vi "map_diag_piastre.vi"() -> ()   [LabVIEW 2015]
panel:
  in  "z inizio":bool
  in  "y inizio":bool
  in  "Positioning Done":bool
  in  "x inizio":bool
  in  "y inizio":bool
  in  "Positioning Done":bool
  in  "y inizio":bool
  in  "Positioning Done":bool
  in  "KILL":bool
  in  "PAUSE":bool
  in  "RESUME":bool
  in  "QUIT":bool
  in  "Positioning Done":bool
  in  "y inizio":bool
  in  "x inizio":bool
  in  "End":bool
  in  "zero z - end":bool
  in  "zero x - end":bool
  in  "zero y - end":bool
  out "output":string
  out "command":string
  in  "zero done":bool
  in  "zero z":bool
  in  "zero x":bool
  in  "zero y":bool
  # "Comandi di emergenza"
  # "Posiziono in zero"
  # "Vado al punto di partenza\nDiagonale Left Internal"
  # "Vado al punto di partenza\nDiagonale Right Internal"
  # "Vado al punto di partenza\nDiagonale Left External"
  # "Vado al punto di partenza\nDiagonale Right External"
  # "Ritorno a zero"
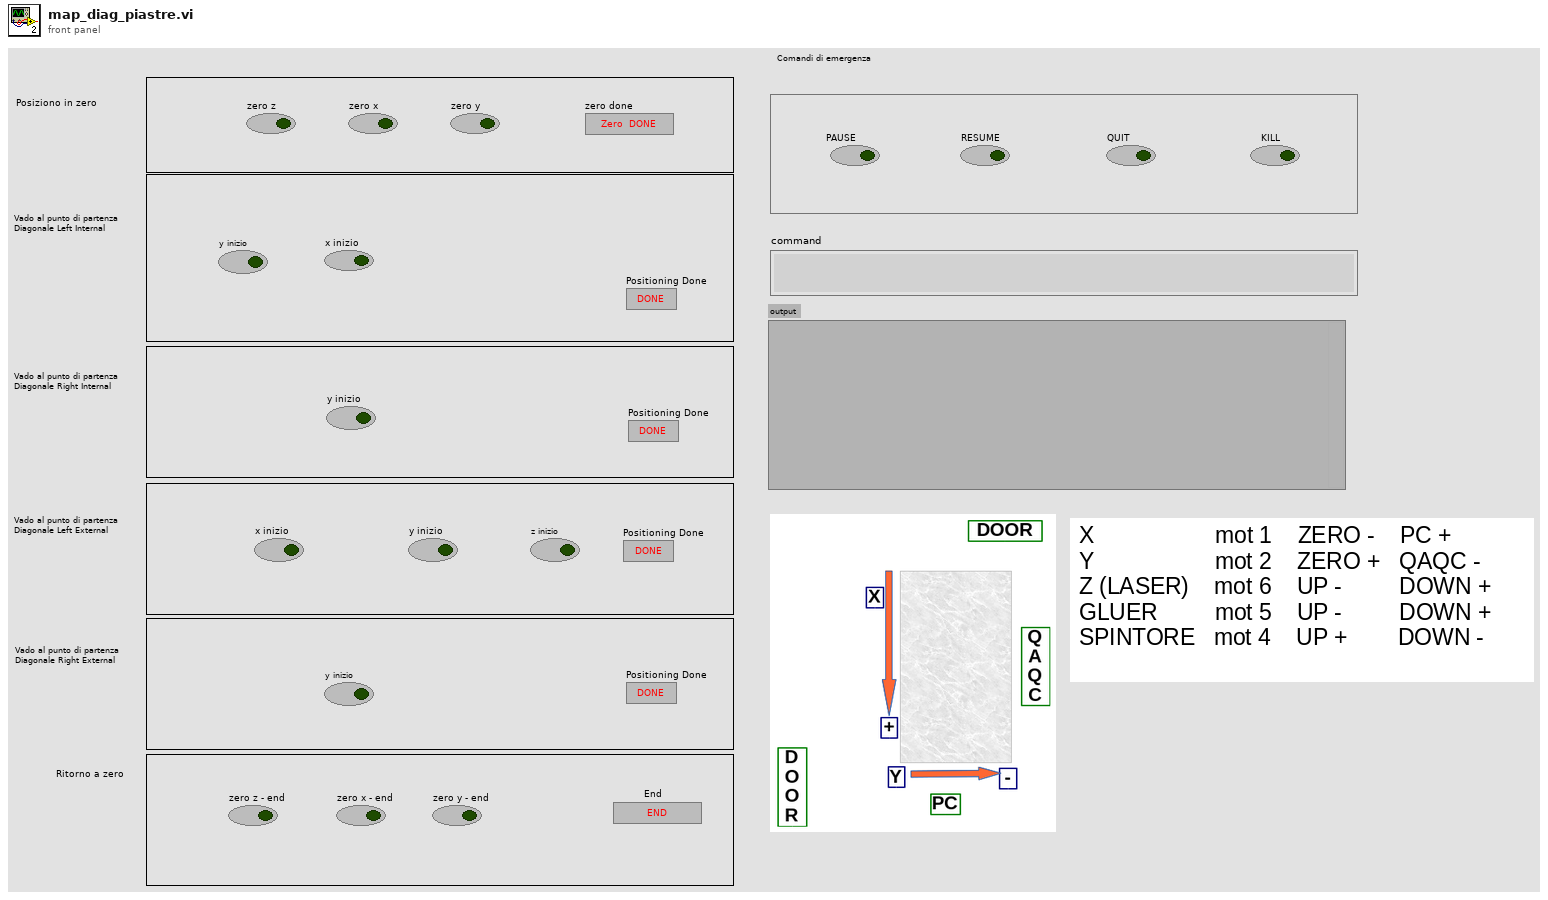
[diagram p1: front panel]
types:
  T1 = enum16{"open", "replace", "create", "open or create", "replace or create", "replace or create with confirmation"}
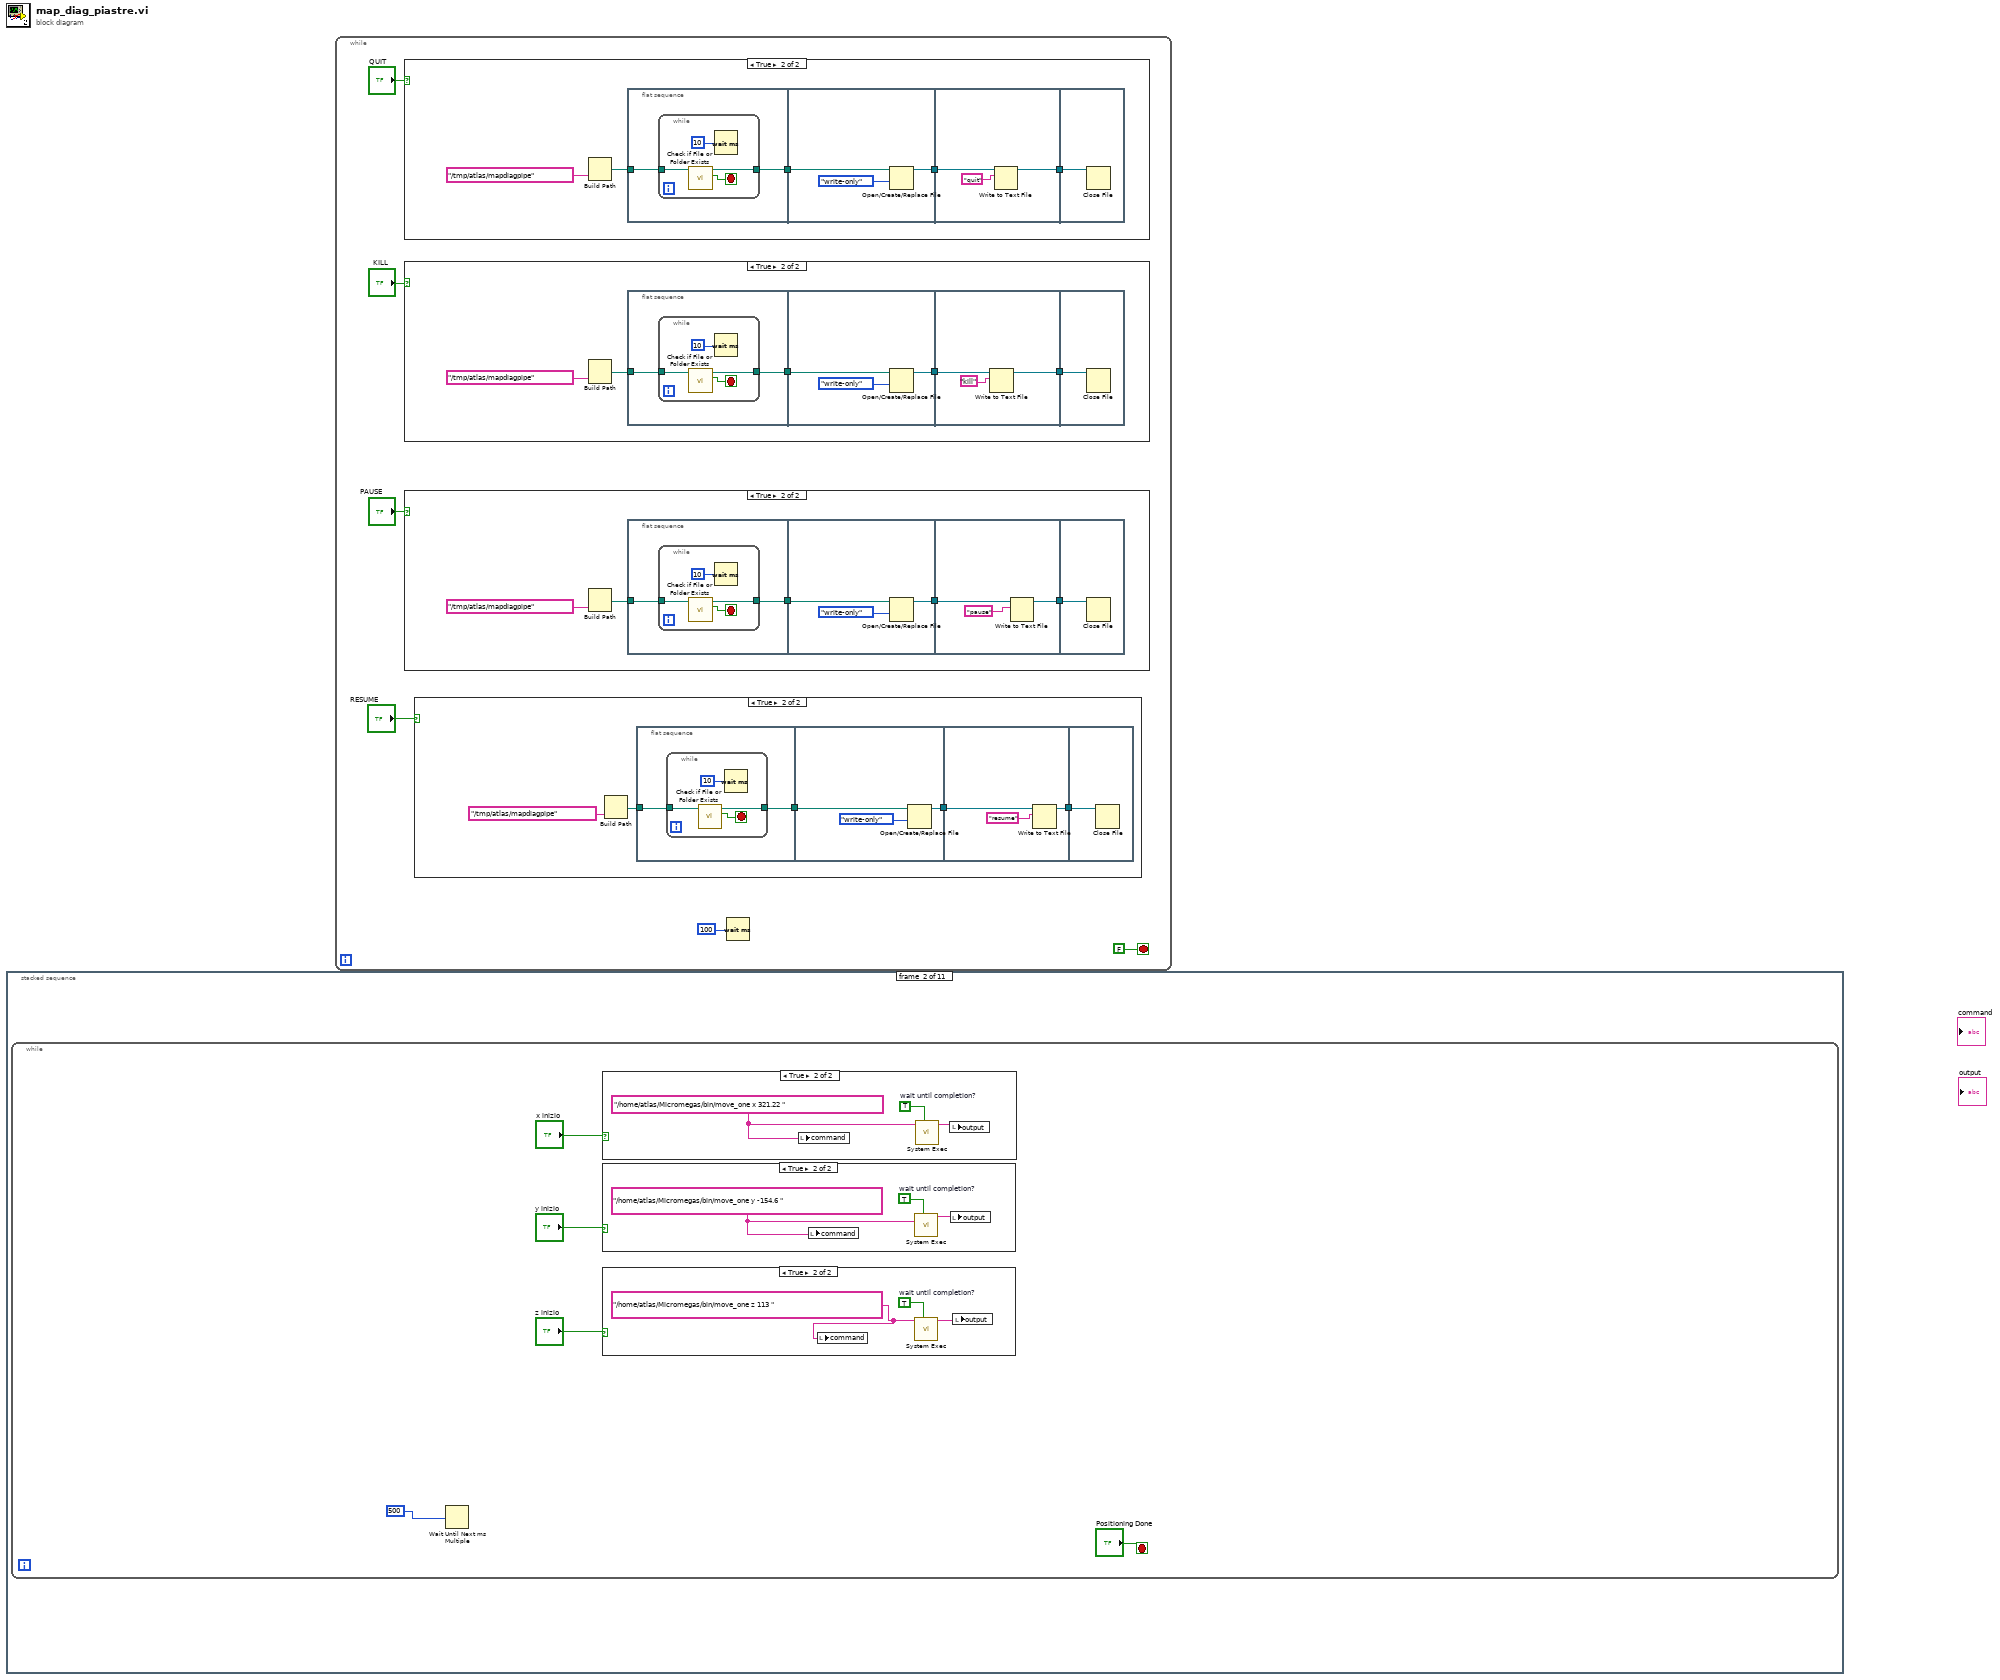
[diagram p0: block diagram]
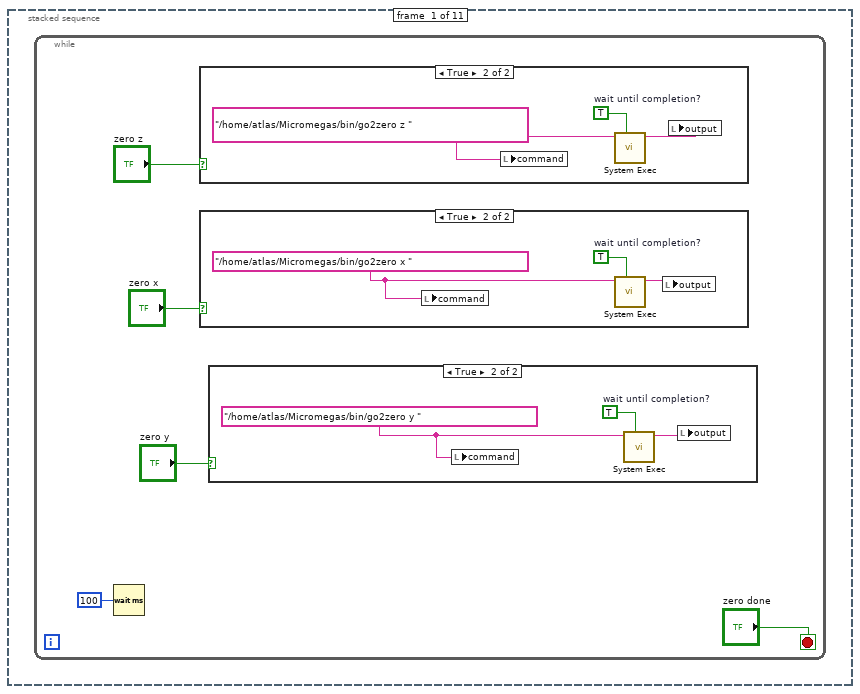
[diagram p6: hidden frame]
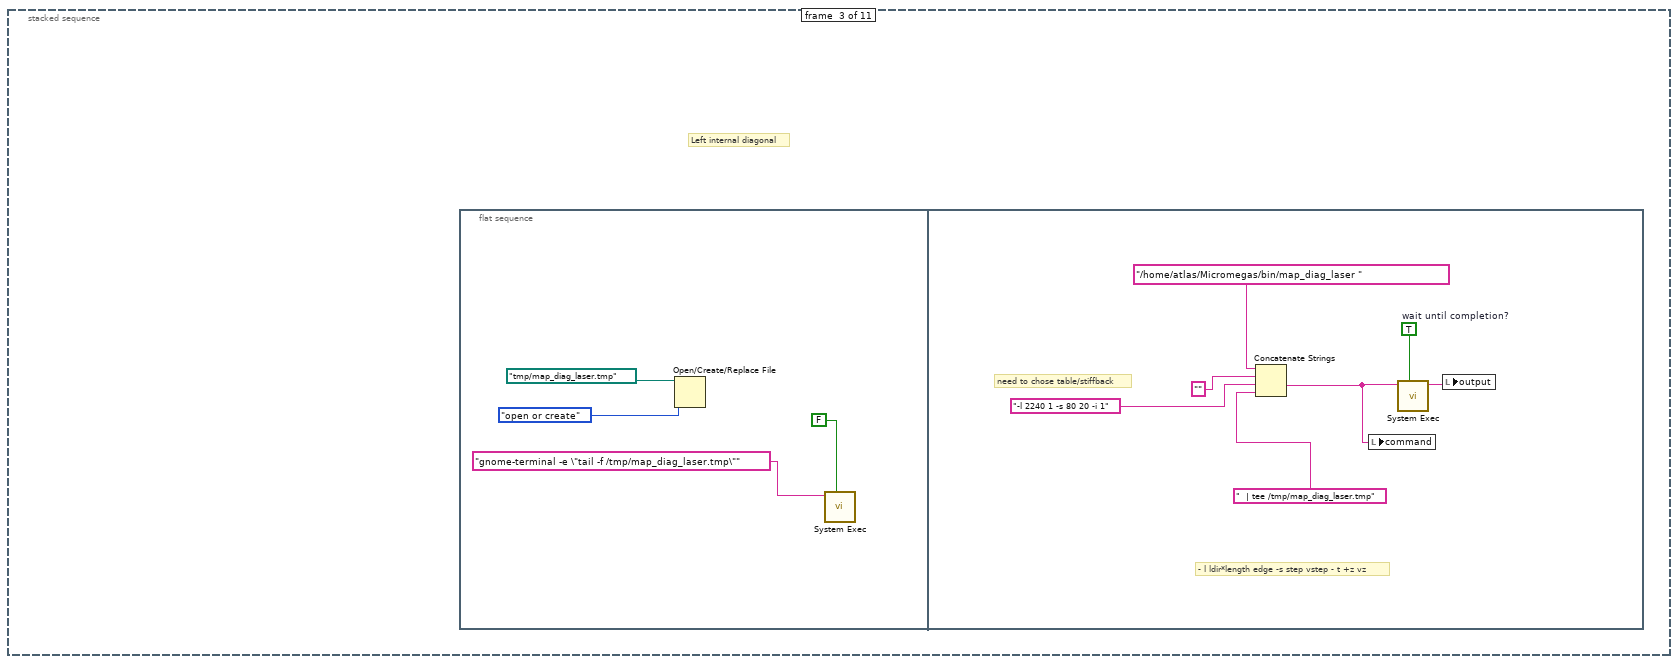
[diagram p13: hidden frame]
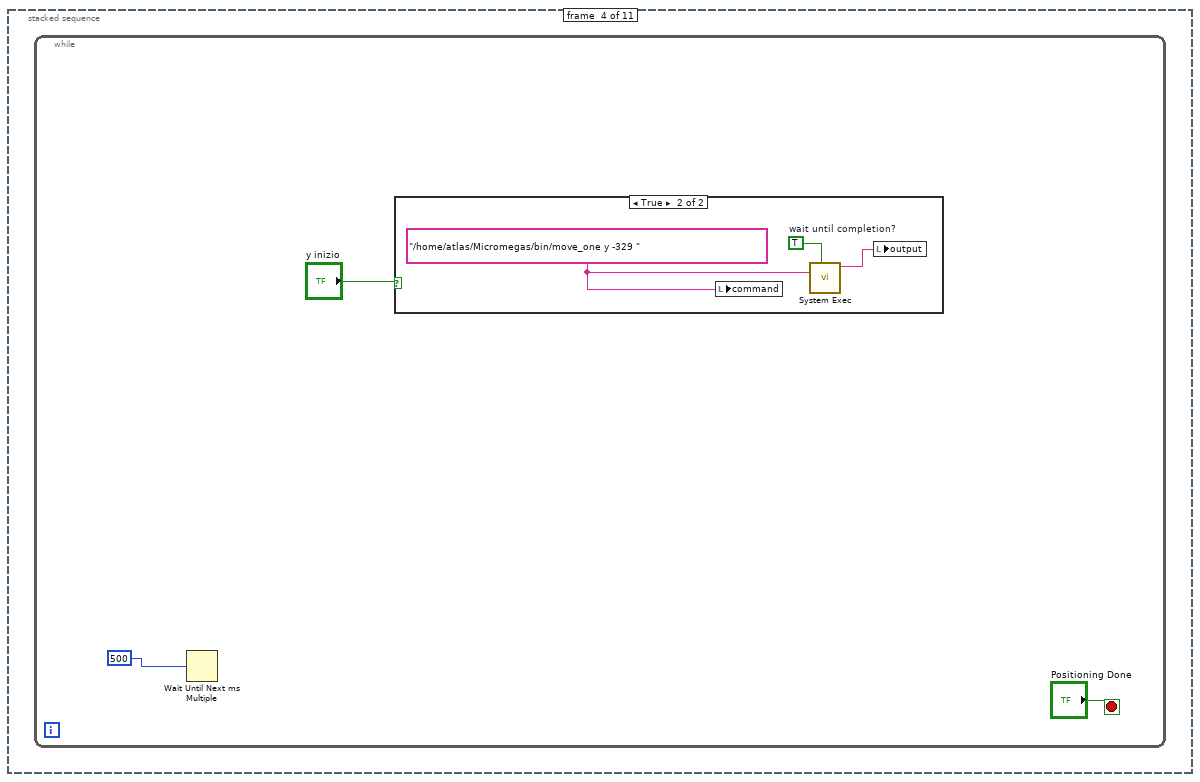
[diagram p14: hidden frame]
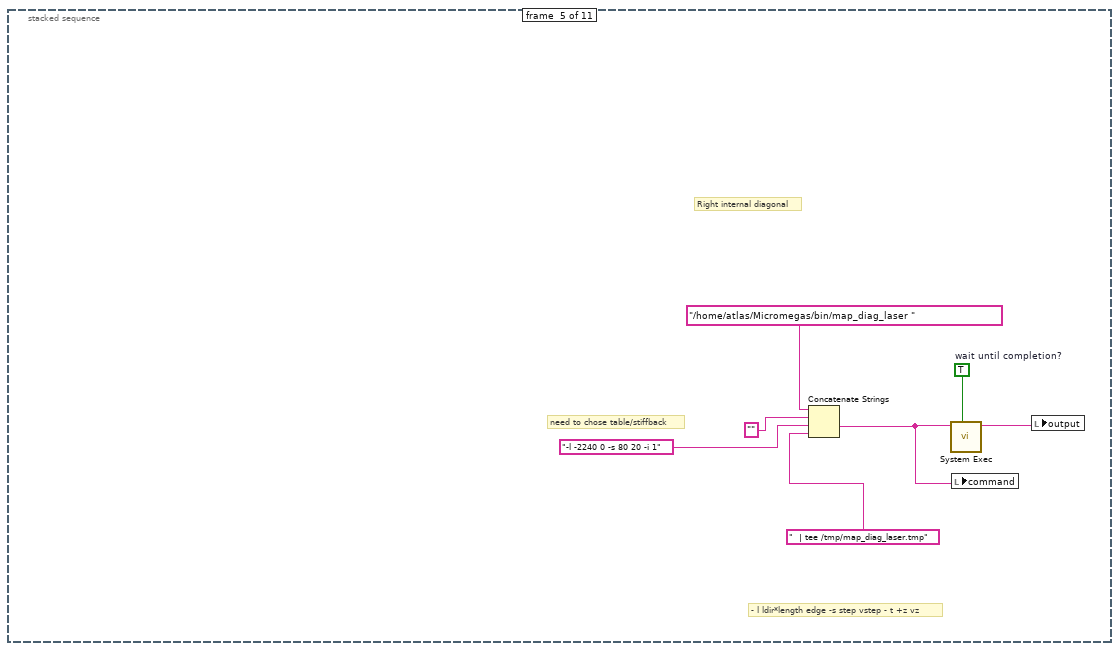
[diagram p16: hidden frame]
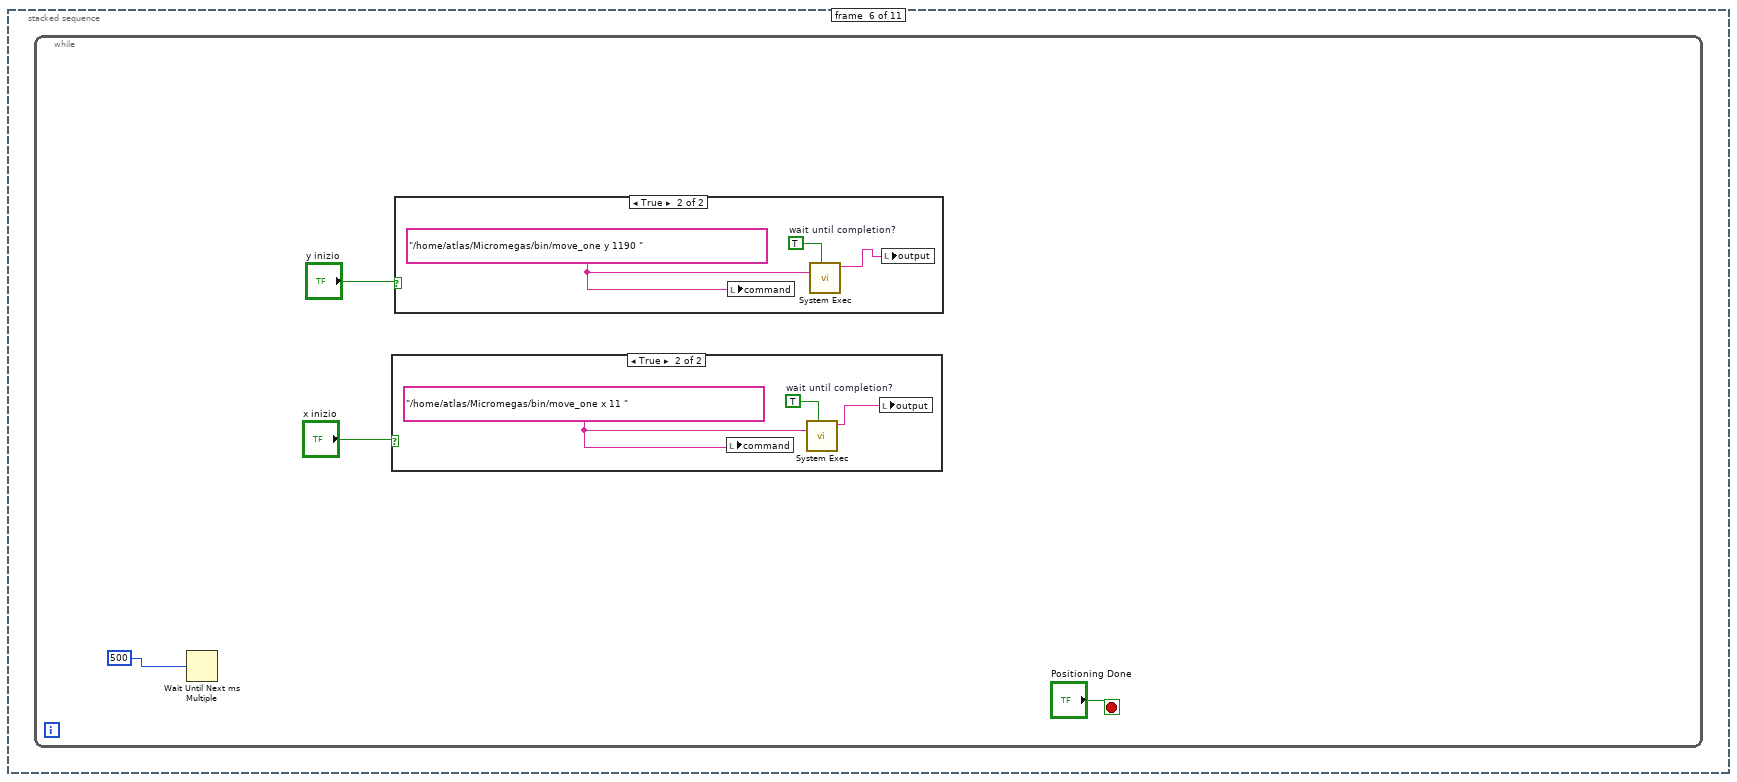
[diagram p17: hidden frame]
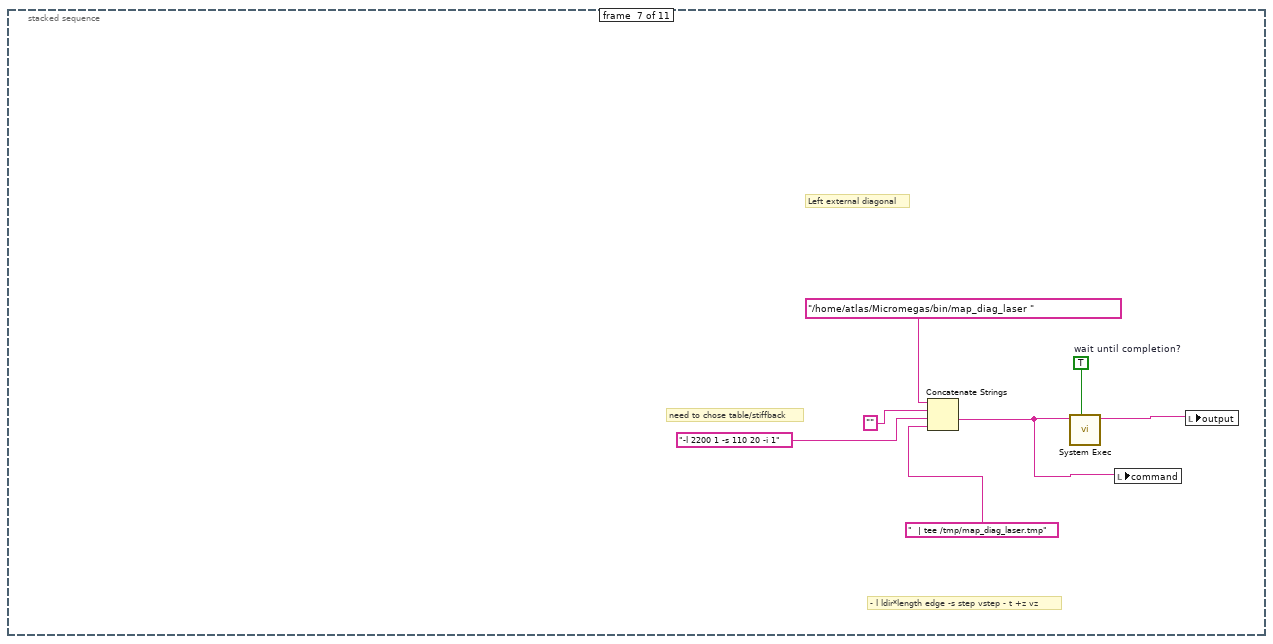
[diagram p20: hidden frame]
diagram:
  n1 = stacked-sequence {
    frame #0 {
      n2 = while {
        stop <- "zero done" stop-if-true
        n3 = Wait (ms)(milliseconds to wait=u32 100) -> ()  [unwired: 1 out]
        n4 = case shown="True" "zero z" {
          frame False {
          }
          frame True {
            w13 = "/home/atlas/Micromegas/bin/go2zero z " ("string")
            w14 = TRUE  # wait until completion?
            n5 = local write "command"(w13) -> ()
            n6 = call <vilib>:"System Exec.vi"("wait until completion? (T)"=w14, "command line"=w13) -> ("standard output"=w12:string)  [unwired: 6 in, 3 out]
            n7 = local write "output"(w12) -> ()
          }
        }
        n8 = case shown="True" "zero x" {
          frame False {
          }
          frame True {
            w10 = "/home/atlas/Micromegas/bin/go2zero x " ("string")
            w11 = TRUE  # wait until completion?
            n9 = local write "command"(w10) -> ()
            n10 = call <vilib>:"System Exec.vi"("wait until completion? (T)"=w11, "command line"=w10) -> ("standard output"=w9:string)  [unwired: 6 in, 3 out]
            n11 = local write "output"(w9) -> ()
          }
        }
        n12 = case shown="True" "zero y" {
          frame False {
          }
          frame True {
            w7 = "/home/atlas/Micromegas/bin/go2zero y " ("string")
            w8 = TRUE  # wait until completion?
            n13 = local write "command"(w7) -> ()
            n14 = call <vilib>:"System Exec.vi"("wait until completion? (T)"=w8, "command line"=w7) -> ("standard output"=w6:string)  [unwired: 6 in, 3 out]
            n15 = local write "output"(w6) -> ()
          }
        }
      }
    }
    frame #1 {
      n16 = while {
        stop <- "Positioning Done" stop-if-true
        n17 = Wait Until Next ms Multiple(millisecond multiple=u32 500 ("millisecond timer value")) -> ()  [unwired: 1 out]
        n18 = case shown="True" "y inizio" {
          frame False {
          }
          frame True {
            w23 = "/home/atlas/Micromegas/bin/move_one y -154.6 " ("string")
            w25 = TRUE  # wait until completion?
            n19 = local write "command"(w23) -> ()
            n20 = call <vilib>:"System Exec.vi"("wait until completion? (T)"=w25, "command line"=w23) -> ("standard output"=w24:string)  [unwired: 6 in, 3 out]
            n21 = local write "output"(w24) -> ()
          }
        }
        n22 = case shown="True" "z inizio" {
          frame False {
          }
          frame True {
            w20 = "/home/atlas/Micromegas/bin/move_one z 113 " ("string")
            w22 = TRUE  # wait until completion?
            n23 = local write "command"(w20) -> ()
            n24 = call <vilib>:"System Exec.vi"("wait until completion? (T)"=w22, "command line"=w20) -> ("standard output"=w21:string)  [unwired: 6 in, 3 out]
            n25 = local write "output"(w21) -> ()
          }
        }
        n26 = case shown="True" "x inizio" {
          frame False {
          }
          frame True {
            w26 = "/home/atlas/Micromegas/bin/move_one x 321.22 " ("string")
            w28 = TRUE  # wait until completion?
            n27 = local write "command"(w26) -> ()
            n28 = call <vilib>:"System Exec.vi"("wait until completion? (T)"=w28, "command line"=w26) -> ("standard output"=w27:string)  [unwired: 6 in, 3 out]
            n29 = local write "output"(w27) -> ()
          }
        }
      }
    }
    frame #2 {
      # "Left internal diagonal"
      n30 = flat-sequence {
        frame #0 {
          n31 = Open/Create/Replace File(file path (use dialog)=path "/tmp/map_diag_laser.tmp", operation (0:open)=T1."open or create") -> ()  [unwired: 4 in, 3 out]
          n32 = call <vilib>:"System Exec.vi"("wait until completion? (T)"=FALSE, "command line"="gnome-terminal -e \"tail -f /tmp/map_diag_laser.tmp\"") -> ()  [unwired: 6 in, 4 out]
        }
        frame #1 {
          w39 = TRUE  # wait until completion?
          # "need to chose table/stiffback"
          # "- l ldir*length edge -s step vstep - t +z vz"
          n33 = Concatenate Strings("/home/atlas/Micromegas/bin/map_diag_laser " ("string"), "" ("string"), "-l 2240 1 -s 80 20 -i 1" ("string"), "  | tee /tmp/map_diag_laser.tmp" ("string")) -> (w36:string)
          n34 = local write "command"(w36) -> ()
          n35 = call <vilib>:"System Exec.vi"("wait until completion? (T)"=w39, "command line"=w36) -> ("standard output"=w37:string)  [unwired: 6 in, 3 out]
          n36 = local write "output"(w37) -> ()
        }
      }
    }
    frame #3 {
      n37 = while {
        stop <- "Positioning Done" stop-if-true
        n38 = Wait Until Next ms Multiple(millisecond multiple=u32 500 ("millisecond timer value")) -> ()  [unwired: 1 out]
        n39 = case shown="True" "y inizio" {
          frame False {
          }
          frame True {
            w43 = "/home/atlas/Micromegas/bin/move_one y -329 " ("string")
            w45 = TRUE  # wait until completion?
            n40 = local write "command"(w43) -> ()
            n41 = call <vilib>:"System Exec.vi"("wait until completion? (T)"=w45, "command line"=w43) -> ("standard output"=w44:string)  [unwired: 6 in, 3 out]
            n42 = local write "output"(w44) -> ()
          }
        }
      }
    }
    frame #4 {
      w52 = TRUE  # wait until completion?
      # "Right internal diagonal"
      # "need to chose table/stiffback"
      # "- l ldir*length edge -s step vstep - t +z vz"
      n43 = Concatenate Strings("/home/atlas/Micromegas/bin/map_diag_laser " ("string"), "" ("string"), "-l -2240 0 -s 80 20 -i 1" ("string"), "  | tee /tmp/map_diag_laser.tmp" ("string")) -> (w46:string)
      n44 = call <vilib>:"System Exec.vi"("wait until completion? (T)"=w52, "command line"=w46) -> ("standard output"=w47:string)  [unwired: 6 in, 3 out]
      n45 = local write "command"(w46) -> ()
      n46 = local write "output"(w47) -> ()
    }
    frame #5 {
      n47 = while {
        stop <- "Positioning Done" stop-if-true
        n48 = Wait Until Next ms Multiple(millisecond multiple=u32 500 ("millisecond timer value")) -> ()  [unwired: 1 out]
        n49 = case shown="True" "x inizio" {
          frame False {
          }
          frame True {
            w57 = "/home/atlas/Micromegas/bin/move_one x 11 " ("string")
            w59 = TRUE  # wait until completion?
            n50 = local write "command"(w57) -> ()
            n51 = call <vilib>:"System Exec.vi"("wait until completion? (T)"=w59, "command line"=w57) -> ("standard output"=w58:string)  [unwired: 6 in, 3 out]
            n52 = local write "output"(w58) -> ()
          }
        }
        n53 = case shown="True" "y inizio" {
          frame False {
          }
          frame True {
            w60 = "/home/atlas/Micromegas/bin/move_one y 1190 " ("string")
            w62 = TRUE  # wait until completion?
            n54 = local write "command"(w60) -> ()
            n55 = call <vilib>:"System Exec.vi"("wait until completion? (T)"=w62, "command line"=w60) -> ("standard output"=w61:string)  [unwired: 6 in, 3 out]
            n56 = local write "output"(w61) -> ()
          }
        }
      }
    }
    frame #6 {
      w69 = TRUE  # wait until completion?
      # "Left external diagonal"
      # "need to chose table/stiffback"
      # "- l ldir*length edge -s step vstep - t +z vz"
      n57 = Concatenate Strings("/home/atlas/Micromegas/bin/map_diag_laser " ("string"), "" ("string"), "-l 2200 1 -s 110 20 -i 1" ("string"), "  | tee /tmp/map_diag_laser.tmp" ("string")) -> (w63:string)
      n58 = call <vilib>:"System Exec.vi"("wait until completion? (T)"=w69, "command line"=w63) -> ("standard output"=w64:string)  [unwired: 6 in, 3 out]
      n59 = local write "command"(w63) -> ()
      n60 = local write "output"(w64) -> ()
    }
    frame #7 {
      n61 = while {
        stop <- "Positioning Done" stop-if-true
        n62 = Wait Until Next ms Multiple(millisecond multiple=u32 500 ("millisecond timer value")) -> ()  [unwired: 1 out]
        n63 = case shown="True" "y inizio" {
          frame False {
          }
          frame True {
            w73 = "/home/atlas/Micromegas/bin/move_one y -505 " ("string")
            w75 = TRUE  # wait until completion?
            n64 = local write "command"(w73) -> ()
            n65 = call <vilib>:"System Exec.vi"("wait until completion? (T)"=w75, "command line"=w73) -> ("standard output"=w74:string)  [unwired: 6 in, 3 out]
            n66 = local write "output"(w74) -> ()
          }
        }
      }
    }
    frame #8 {
      w82 = TRUE  # wait until completion?
      # "Right external diagonal"
      # "need to chose table/stiffback"
      # "- l ldir*length edge -s step vstep - t +z vz"
      n67 = Concatenate Strings("/home/atlas/Micromegas/bin/map_diag_laser " ("string"), "" ("string"), "-l -2200 0 -s 110 20 -i 1" ("string"), "  | tee /tmp/map_diag_laser.tmp" ("string")) -> (w76:string)
      n68 = call <vilib>:"System Exec.vi"("wait until completion? (T)"=w82, "command line"=w76) -> ("standard output"=w77:string)  [unwired: 6 in, 3 out]
      n69 = local write "command"(w76) -> ()
      n70 = local write "output"(w77) -> ()
    }
    frame #9 {
      n71 = while {
        stop <- "End" stop-if-true
        n72 = Wait (ms)(milliseconds to wait=u32 100) -> ()  [unwired: 1 out]
        n73 = case shown="True" "zero z - end" {
          frame False {
          }
          frame True {
            w95 = "/home/atlas/Micromegas/bin/go2zero z " ("string")
            w96 = TRUE  # wait until completion?
            n74 = local write "command"(w95) -> ()
            n75 = call <vilib>:"System Exec.vi"("wait until completion? (T)"=w96, "command line"=w95) -> ("standard output"=w94:string)  [unwired: 6 in, 3 out]
            n76 = local write "output"(w94) -> ()
          }
        }
        n77 = case shown="True" "zero x - end" {
          frame False {
          }
          frame True {
            w92 = "/home/atlas/Micromegas/bin/go2zero x " ("string")
            w93 = TRUE  # wait until completion?
            n78 = local write "command"(w92) -> ()
            n79 = call <vilib>:"System Exec.vi"("wait until completion? (T)"=w93, "command line"=w92) -> ("standard output"=w91:string)  [unwired: 6 in, 3 out]
            n80 = local write "output"(w91) -> ()
          }
        }
        n81 = case shown="True" "zero y - end" {
          frame False {
          }
          frame True {
            w89 = "/home/atlas/Micromegas/bin/go2zero y " ("string")
            w90 = TRUE  # wait until completion?
            n82 = local write "command"(w89) -> ()
            n83 = call <vilib>:"System Exec.vi"("wait until completion? (T)"=w90, "command line"=w89) -> ("standard output"=w88:string)  [unwired: 6 in, 3 out]
            n84 = local write "output"(w88) -> ()
          }
        }
      }
    }
    frame #10 {
      n85 = One Button Dialog(message="Per comodita`, rinominare il file (non verra` comunque sovrascritto)") -> ()  [unwired: 1 in, 1 out]
    }
  }
  n86 = while {
    stop <- FALSE stop-if-true
    n87 = case shown="True" "QUIT" {
      frame False {
      }
      frame True {
        n88 = Build Path(name or relative path="/tmp/atlas/mapdiagpipe" ("string")) -> (appended path=w158:path)  [unwired: 1 in]
        n89 = flat-sequence {
          tunnel: [w164] -> w162
          tunnel: w158 -> [w163]
          tunnel: w162 -> [w171]
          tunnel: [w169] -> w161
          tunnel: w161 -> [w174]
          tunnel: [w173] -> w160
          tunnel: w160 -> [w175]
          frame #0 {
            n90 = while {
              tunnel: [w166] -> w164
              tunnel: w163 -> [w165]
              stop <- w167 stop-if-true
              n91 = call <vilib>:"Check if File or Folder Exists.vi"("path"=w165) -> ("file or folder exists?"=w167:bool, "dup path"=w166:path)  [unwired: 8 in, 1 out]
              n92 = Wait (ms)(milliseconds to wait=u32 10) -> ()  [unwired: 1 out]
            }
          }
          frame #1 {
            n93 = Open/Create/Replace File(file path (use dialog)=w171, access (0:read/write)=enum16{"read/write", "read-only", "write-only"}."write-only") -> (refnum out=w169:refnum<file>)  [unwired: 4 in, 2 out]
          }
          frame #2 {
            n94 = Write to Text File(file (use dialog)=w174, text="quit") -> (refnum out=w173:refnum<file>)  [unwired: 2 in, 2 out]
          }
          frame #3 {
            n95 = Close File(refnum=w175) -> ()  [unwired: 1 in, 2 out]
          }
        }
      }
    }
    n96 = case shown="True" "KILL" {
      frame False {
      }
      frame True {
        n97 = Build Path(name or relative path="/tmp/atlas/mapdiagpipe" ("string")) -> (appended path=w122:path)  [unwired: 1 in]
        n98 = flat-sequence {
          tunnel: [w128] -> w126
          tunnel: w122 -> [w127]
          tunnel: w126 -> [w135]
          tunnel: [w133] -> w125
          tunnel: w125 -> [w138]
          tunnel: [w137] -> w124
          tunnel: w124 -> [w139]
          frame #0 {
            n99 = while {
              tunnel: [w130] -> w128
              tunnel: w127 -> [w129]
              stop <- w131 stop-if-true
              n100 = call <vilib>:"Check if File or Folder Exists.vi"("path"=w129) -> ("file or folder exists?"=w131:bool, "dup path"=w130:path)  [unwired: 8 in, 1 out]
              n101 = Wait (ms)(milliseconds to wait=u32 10) -> ()  [unwired: 1 out]
            }
          }
          frame #1 {
            n102 = Open/Create/Replace File(file path (use dialog)=w135, access (0:read/write)=enum16{"read/write", "read-only", "write-only"}."write-only") -> (refnum out=w133:refnum<file>)  [unwired: 4 in, 2 out]
          }
          frame #2 {
            n103 = Write to Text File(file (use dialog)=w138, text="kill") -> (refnum out=w137:refnum<file>)  [unwired: 2 in, 2 out]
          }
          frame #3 {
            n104 = Close File(refnum=w139) -> ()  [unwired: 1 in, 2 out]
          }
        }
      }
    }
    n105 = case shown="True" "PAUSE" {
      frame False {
      }
      frame True {
        n106 = Build Path(name or relative path="/tmp/atlas/mapdiagpipe" ("string")) -> (appended path=w104:path)  [unwired: 1 in]
        n107 = flat-sequence {
          tunnel: [w110] -> w108
          tunnel: w104 -> [w109]
          tunnel: w108 -> [w117]
          tunnel: [w115] -> w107
          tunnel: w107 -> [w120]
          tunnel: [w119] -> w106
          tunnel: w106 -> [w121]
          frame #0 {
            n108 = while {
              tunnel: [w112] -> w110
              tunnel: w109 -> [w111]
              stop <- w113 stop-if-true
              n109 = call <vilib>:"Check if File or Folder Exists.vi"("path"=w111) -> ("file or folder exists?"=w113:bool, "dup path"=w112:path)  [unwired: 8 in, 1 out]
              n110 = Wait (ms)(milliseconds to wait=u32 10) -> ()  [unwired: 1 out]
            }
          }
          frame #1 {
            n111 = Open/Create/Replace File(file path (use dialog)=w117, access (0:read/write)=enum16{"read/write", "read-only", "write-only"}."write-only") -> (refnum out=w115:refnum<file>)  [unwired: 4 in, 2 out]
          }
          frame #2 {
            n112 = Write to Text File(file (use dialog)=w120, text="pause") -> (refnum out=w119:refnum<file>)  [unwired: 2 in, 2 out]
          }
          frame #3 {
            n113 = Close File(refnum=w121) -> ()  [unwired: 1 in, 2 out]
          }
        }
      }
    }
    n114 = case shown="True" "RESUME" {
      frame False {
      }
      frame True {
        n115 = Build Path(name or relative path="/tmp/atlas/mapdiagpipe" ("string")) -> (appended path=w140:path)  [unwired: 1 in]
        n116 = flat-sequence {
          tunnel: [w146] -> w144
          tunnel: w140 -> [w145]
          tunnel: w144 -> [w153]
          tunnel: [w151] -> w143
          tunnel: w143 -> [w156]
          tunnel: [w155] -> w142
          tunnel: w142 -> [w157]
          frame #0 {
            n117 = while {
              tunnel: [w148] -> w146
              tunnel: w145 -> [w147]
              stop <- w149 stop-if-true
              n118 = call <vilib>:"Check if File or Folder Exists.vi"("path"=w147) -> ("file or folder exists?"=w149:bool, "dup path"=w148:path)  [unwired: 8 in, 1 out]
              n119 = Wait (ms)(milliseconds to wait=u32 10) -> ()  [unwired: 1 out]
            }
          }
          frame #1 {
            n120 = Open/Create/Replace File(file path (use dialog)=w153, access (0:read/write)=enum16{"read/write", "read-only", "write-only"}."write-only") -> (refnum out=w151:refnum<file>)  [unwired: 4 in, 2 out]
          }
          frame #2 {
            n121 = Write to Text File(file (use dialog)=w156, text="resume") -> (refnum out=w155:refnum<file>)  [unwired: 2 in, 2 out]
          }
          frame #3 {
            n122 = Close File(refnum=w157) -> ()  [unwired: 1 in, 2 out]
          }
        }
      }
    }
    n123 = Wait (ms)(milliseconds to wait=100) -> ()  [unwired: 1 out]
  }
